vi "initialize file property tag list.vi"(8 "error in":errorcluster, 10 "Line":T1, 11 "engine configuration in":refnum<class "engine configuration.lvclass">) -> (0 "error out":errorcluster, 1 "Value":i32, 2 "Item Names":string[](array[string]))   [LabVIEW 2015, in "TDMS datalogger editor node.lvclass"]
uses:
  TDMS datalogger editor node.lvclass
  <vilib>/NI/Tag Bus Module Framework/channel/TBM channel.lvclass
  <vilib>/NI/Module Execution Interface/Engine Configuration/engine configuration.lvclass
  <vilib>/NI/Tag Bus/tag/Data Type.ctl
  <vilib>/NI/Tag Bus/tag/tag descriptor.lvclass/tag descriptor.ctl
  <vilib>/NI/Tag Bus Module Framework/channel/TBM channel.lvclass/TBM channel.ctl
  <vilib>/NI/Tag Bus/tag/write data type.vi
  <vilib>/NI/Tag Bus Module Framework/channel/Write channel classification.vi
  <vilib>/NI/Tag Bus/tag/tag descriptor.lvclass
  module/configuration/TDMS datalogger configuration.lvclass
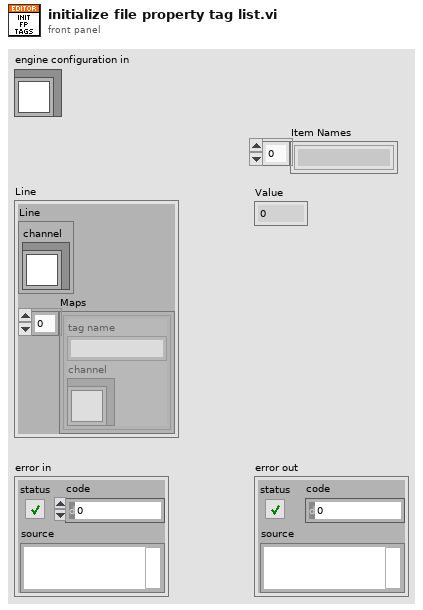
[diagram p1: front panel]
types:
  T1 = cluster{"Line":cluster{"channel":refnum<class "TBM channel.lvclass">}, "Maps":cluster{"tag name":string, "channel":refnum<class "TBM channel.lvclass">}[]}
  T2 = typedef "tag bus.lvlib/tag descriptor.lvclass/Data Type.ctl" = enum16{"Double", "Single", "I64", "I32", "I16", "I8", "U64", "U32", "U16", "U8", "Boolean", "String", "Array of Double", "Array of Single", "Array of I64", "Array of I32", "Array of I16", "Array of I8", "Array of U64", "Array of U32", "Array of U16", "Array of U8", "Array of Boolean", "Array of String"}
  T3 = cluster{"tag name":string, "channel":refnum<class "TBM channel.lvclass">}[]
  T4 = typedef "TBM channel.lvclass/channel classification.ctl" = enum16{"input data", "output data", "processing parameter", "processing result"}
  T5 = cluster{"tag name":string, "channel":refnum<class "TBM channel.lvclass">}
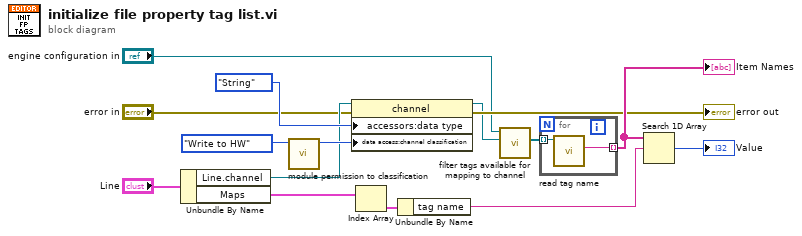
[diagram p0: block diagram]
diagram:
  n1 = Unbundle By Name("Line") -> ("Line.channel"=w5:refnum<class "TBM channel.lvclass">, "Maps"=w12:T3)
  n2 = call "module permission to classification.vi"("view direction"=enum32{"Read from HW", "Write to HW"}."Write to HW" ("Access Type")) -> ("channel classification"=w13:T4)  [unwired: 10 in]
  n3 = property class="channel"(reference=w5, error in="error in", "accessors:data type"=Data_Type."String" ("data type"), "data access:channel classification"=w13) -> (reference out=w6:refnum<class "TBM channel.lvclass">, error out=→"error out":errorcluster)
  n4 = Index Array(array=w12) -> (element=w10:T5)  [unwired: 1 in]
  n5 = Unbundle By Name(w10) -> ("tag name"=w11:string)
  n6 = call-dynamic "filter tags available for mapping to channel.vi"("channel to map to"=w6, "engine configuration in"="engine configuration in") -> ("filtered tags"=w7:refnum<class "tag descriptor.lvclass">[])  [unwired: 8 in, 1 out]
  n7 = for {
    tunnel: w7 -> [w17] mode=indexing
    tunnel: [w16] -> w9 mode=indexing
    n8 = call <vilib>:"read tag name.vi"("system tag in"=w17) -> ("name"=w16:string)  [unwired: 8 in, 2 out]
  }
  "Item Names" <- w9
  n9 = Search 1D Array(1D array=w9, element=w11) -> (index of element=→"Value":i32)  [unwired: 1 in]
